vi "SynchiIO.PXI4461.SetData.vi"(8 "error in (no error)":errorcluster, 10 "Data In":string, 11 "SynchiIO.PXI4461":refnum<class "SynchiIO.PXI4461.lvclass">) -> (0 "error out":errorcluster, 3 "SynchiIO.PXI4461 out":refnum<class "SynchiIO.PXI4461.lvclass">)   [LabVIEW 2016, in "SynchiIO.PXI4461.lvclass"]
doc: "---------------------------------------------------------------\nJKI State Machine Objects™\nhttp://jki.net/state-machine-objects/\nCopyright (C) 2005-2015, JKI <info@jki.net>\nALL RIGHTS RESERVEDJKI State Machine Objects (SMO) 1.0.0.5\nJKI - JKI\nCopyright (c) 2016, JKI"
uses:
  SynchiIO.PXI4461.lvclass
  SynchiIO.PXI4461.lvclass/SynchiIO.PXI4461.ctl
  Typedefs/DataChanged--EventData--Cluster.ctl
panel:
  # "For instructions on how to use the JKI State Machine Objects, examples and video tutorials, visit:\nhttp://jki.net/state-machine-objects/\n\nJKI State Machine Objects™\nhttp://jki.net/state-machine-objects/\nCopyright (C) 2005-2015, JKI <info@jki.net>\nALL RIGHTS RESERVED"
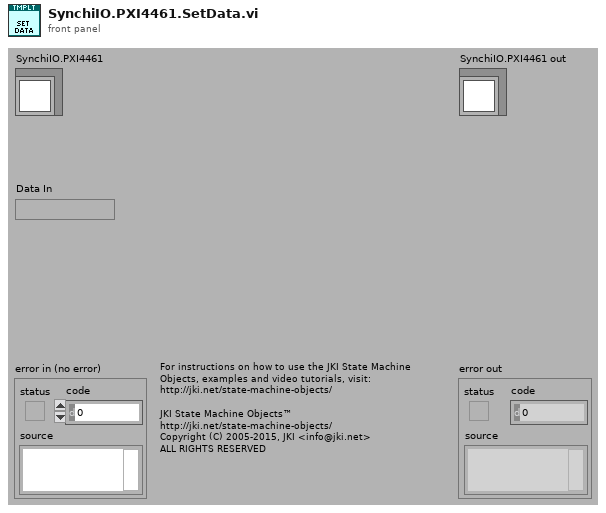
[diagram p1: front panel]
types:
  T1 = typedef "SynchiIO.PXI4461.lvclass/DataChanged--EventData--Cluster.ctl" = cluster{"Timestamp":timestamp, "Old Value":string, "New Value":string}
  T2 = typedef "SynchiIO.PXI4461.lvclass/PrivateData--Ref.ctl" = refnum<data-value>
  T3 = typedef "SynchiIO.PXI4461.lvclass/PrivateData--Cluster.ctl" = cluster{"Configuration":T4, "Public Events":T5, "Protected Events":T6, "Data":string}
  T4 = typedef "SynchiIO.PXI4461.lvclass/Configuration--Cluster.ctl" = cluster{"Suffix":string}
  T5 = typedef "SynchiIO.PXI4461.lvclass/PublicEvents--Cluster.ctl" = cluster{"Data Changed":refnum<user-event>}
  T6 = typedef "SynchiIO.PXI4461.lvclass/ProtectedEvents--Cluster.ctl" = cluster{"API_Template":refnum<user-event>}
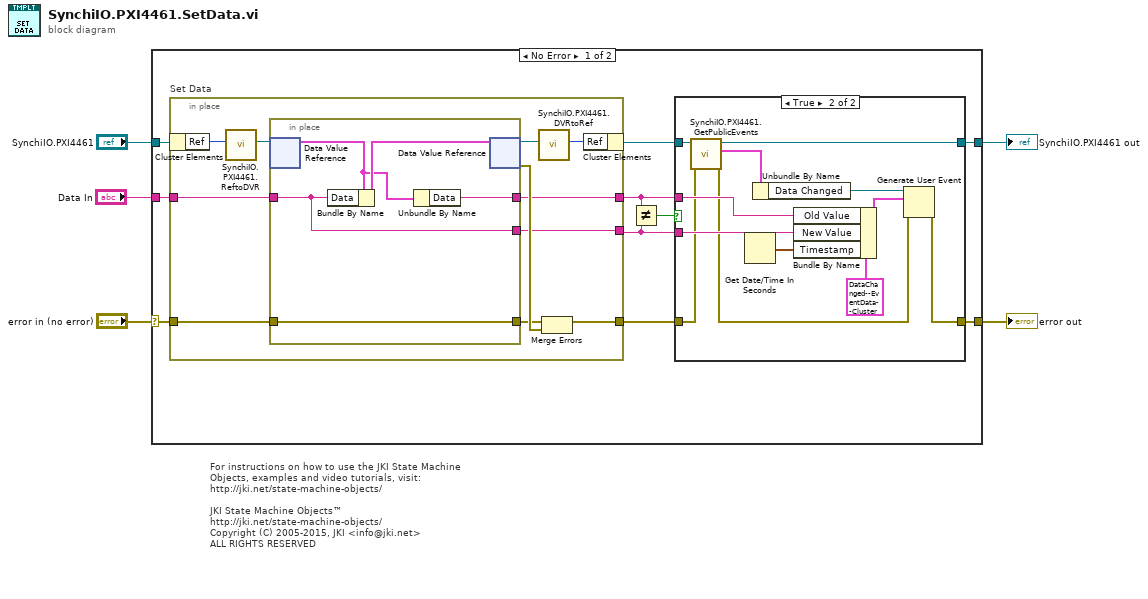
[diagram p0: block diagram]
diagram:
  # "For instructions on how to use the JKI State Machine Objects, examples and video tutorials, visit:\nhttp://jki.net/state-machine-objects/\n\nJKI State Machine Objects™\nhttp://jki.net/state-machine-objects/\nCopyright (C) 2005-2015, JKI <info@jki.net>\nALL RIGHTS RESERVED"
  n1 = case shown="No Error" "error in (no error)" {
    selector: "error in (no error)" -> [w13 w46]
    tunnel: "SynchiIO.PXI4461" -> [w14 w47]
    tunnel: [w11 w46] -> w4
    tunnel: [w6 w47] -> w3
    tunnel: "Data In" -> [w15 _]
    frame No Error {
      n2 = in-place "Set Data" {
        in-place-border: w13 -> [w40]
        in-place-border: [w37] -> w12
        in-place-border: w15 -> [w36]
        in-place-border: [w35] -> w8
        in-place-border: [w34] -> w9
        n3 = in-place-cluster #1(w14) -> ("Ref"=w33:u32)
        n4 = call "SynchiIO.PXI4461.ReftoDVR.vi"("Ref"=w33) -> ("Ref"=w32:T2)  [unwired: 10 in]
        n5 = in-place {
          in-place-border: w40 -> [w45]
          in-place-border: [w45] -> w38
          in-place-border: w36 -> [w43]
          in-place-border: [w43] -> w35
          in-place-border: [w42] -> w34
          n6 = in-place-dvr #2(w32) -> (w41:T3)  [unwired: 1 out]
          n7 = Bundle By Name(cluster=w41, "Data"=w43) -> (w44:T3)
          n8 = Unbundle By Name(w41) -> ("Data"=w42:string)
          n9 = in-place-dvr #2(w44) -> (w31:T2, w39:errorcluster)
        }
        n10 = call "SynchiIO.PXI4461.DVRtoRef.vi"("Ref"=w31) -> ("Ref"=w30:u32)  [unwired: 10 in]
        n11 = Merge Errors(w38, w39) -> (w37:errorcluster)
        n12 = in-place-cluster #1("Ref"=w30) -> (w10:refnum<class "SynchiIO.PXI4461.lvclass">)
      }
      n13 = Not Equal?(x=w9, y=w8) -> (x != y?=w7:bool)
      n14 = case shown="True" w7 {
        tunnel: w12 -> [w16 w21]
        tunnel: w9 -> [_ w26]
        tunnel: w8 -> [_ w25]
        tunnel: [w16 w23] -> w11
        tunnel: w10 -> [w17 w22]
        tunnel: [w17 w19] -> w6
        frame False {
        }
        frame True {
          n15 = call "SynchiIO.PXI4461.GetPublicEvents.vi"("error in (no error)"=w21, "SynchiIO.PXI4461"=w22) -> ("error out"=w20:errorcluster, "SMO.ByRefWithEvents Public Events"=w18:T5, "SynchiIO.PXI4461 out"=w19:refnum<class "SynchiIO.PXI4461.lvclass">)  [unwired: 7 in]
          n16 = Get Date/Time In Seconds() -> (seconds since 1Jan1904=w24:timestamp)
          n17 = Unbundle By Name(w18) -> ("Data Changed"=w29:refnum<user-event>)
          n18 = Bundle By Name(cluster=T1 {"Timestamp"=timestamp(0 s since 1904-01-01), "Old Value"="", "New Value"=""} ("event data"), "Old Value"=w26, "New Value"=w25, "Timestamp"=w24) -> (w27:T1)
          n19 = Generate User Event(user event=w29, event data cluster=w27, error in=w20) -> (error out=w23:errorcluster)  [unwired: 1 in, 1 out]
        }
      }
    }
    frame Error {
    }
  }
  "error out" <- w4
  "SynchiIO.PXI4461 out" <- w3
